vi "AlazarGetChannelnfo.vi"(0 "Handle":u64, 11 "error in (no error)":errorcluster) -> (4 "Handle":u64, 6 "MemorySize_samples":u32, 8 "BitsPerSample":u8, 10 "Return Code":u32, 15 "error out":errorcluster)   [LabVIEW 2009]
doc: "Get the on-board memory in samples per channel, and sample size in bits per sample."
uses:
  ATSApi.dll
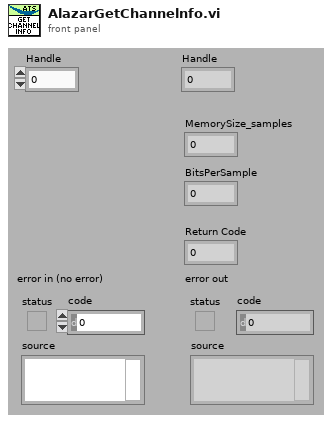
[diagram p1: front panel]
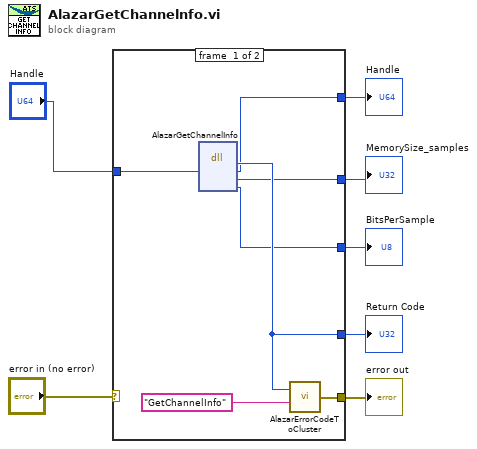
[diagram p0: block diagram]
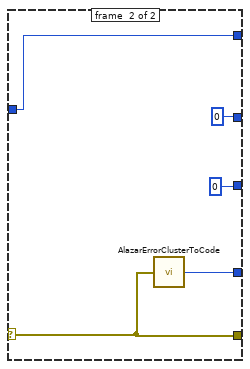
[diagram p2: hidden frame]
diagram:
  n1 = case shown="No Error" "error in (no error)" {
    selector: "error in (no error)" -> [_ w19]
    tunnel: [w11 w19] -> w6
    tunnel: [w13 w18] -> w5
    tunnel: "Handle" -> [w14 w17]
    tunnel: [w10 w17] -> w3
    tunnel: [w9 u32 0] -> w2
    tunnel: [w8 u8 0] -> w1
    frame #0 {
      n2 = dll-call lib="ATSApi.dll" fn="AlazarGetChannelInfo"("handle"=w14) -> ("return type"=w13:u32, "handle"=w10:u64, "memorySizeInSamples"=w9:u32, "bitsPerSample"=w8:u8)  [unwired: 5 in, 2 out]
      n3 = call "AlazarErrorCodeToCluster.vi"("Message"="GetChannelInfo", "Error Code"=w13) -> ("error out"=w11:errorcluster)
    }
    frame #1 {
      n4 = call "AlazarErrorClusterToCode.vi"("error in (no error)"=w19) -> ("Error Code"=w18:u32)
    }
  }
  "Handle" <- w3
  "error out" <- w6
  "Return Code" <- w5
  "MemorySize_samples" <- w2
  "BitsPerSample" <- w1
